vi "Load Scan.vi"(8 "error in (no error)":errorcluster, 9 "File IO.lvclass":refnum<class "File IO.lvclass">, 10 "Reader.lvclass":refnum<class "Reader.lvclass">, 11 "Scanner.lvclass":refnum<class "Scanner.lvclass">) -> (0 "error out":errorcluster, 1 "File IO.lvclass out":refnum<class "File IO.lvclass">, 2 "Reader.lvclass out":refnum<class "Reader.lvclass">, 3 "Scanner.lvclass out":refnum<class "Scanner.lvclass">)   [LabVIEW 2012, in "File IO.lvclass"]
uses:
  File IO.lvclass
  Scanners/Scanner/Scanner.lvclass
  Readers/Reader/Reader.lvclass
  Global/File Locations.vi
  Main/Scan Driver/Settings Panel.vi
  Scanners/Scanner/Write Range UI.vi
  <vilib>/Utility/file.llb/Read From Spreadsheet File (string).vi
  <vilib>/Utility/file.llb/Read From Spreadsheet File (I64).vi
  Readers/Reader/Setup UI.vi
  Main/Scan Driver/Scan Driver.lvclass
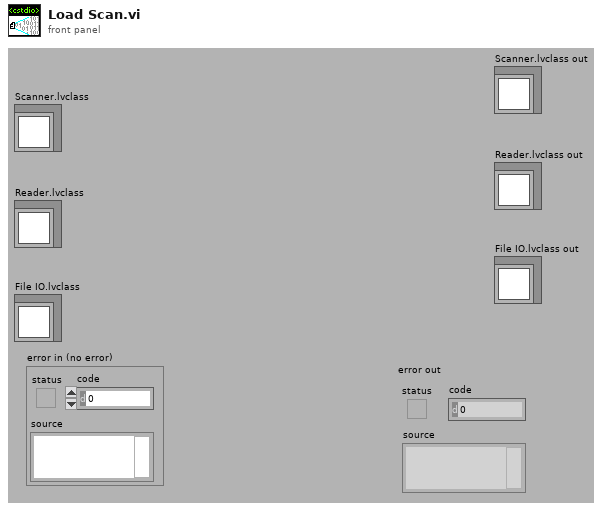
[diagram p1: front panel]
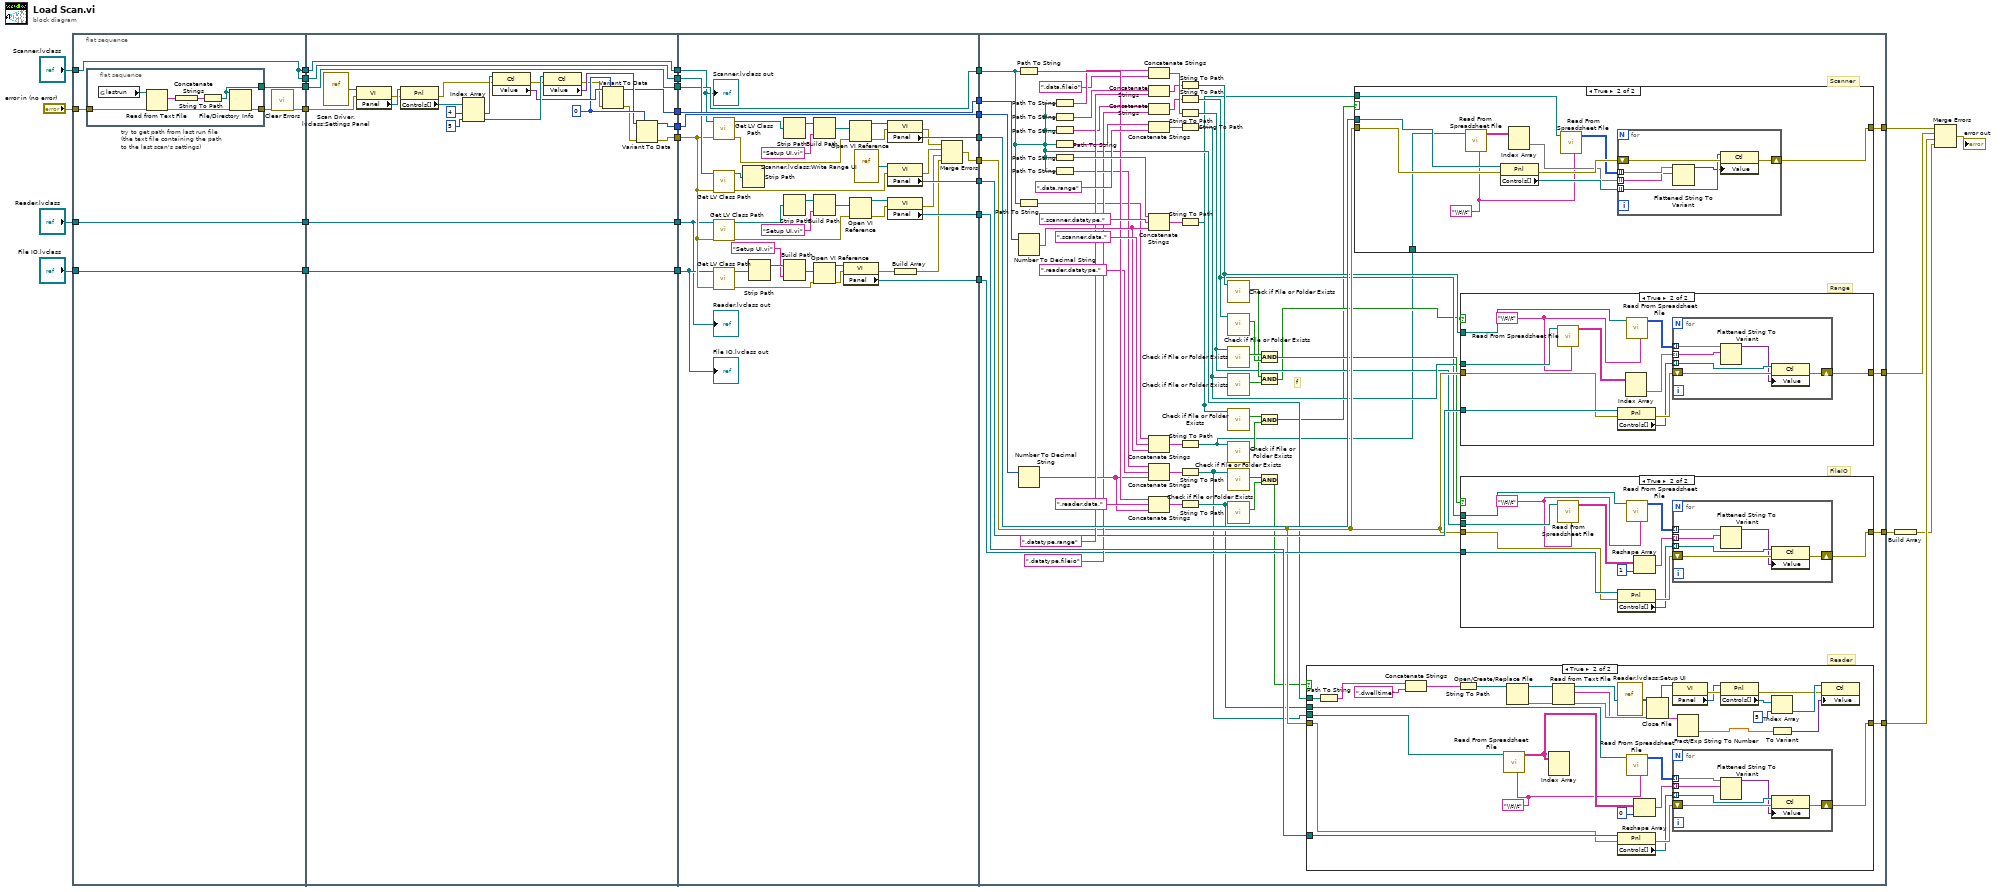
[diagram p0: block diagram]
diagram:
  n1 = flat-sequence {
    tunnel: "Scanner.lvclass" -> [w39]
    tunnel: "error in (no error)" -> [w37]
    tunnel: "Reader.lvclass" -> [w38]
    tunnel: "File IO.lvclass" -> [w33]
    tunnel: [w33] -> w32
    tunnel: [w39] -> w31
    tunnel: [w39] -> w30
    tunnel: [w38] -> w29
    tunnel: [w36] -> w28
    tunnel: [w34] -> w27
    tunnel: w32 -> [w48]
    tunnel: [w48] -> w26
    tunnel: [w70] -> w25
    tunnel: [w69] -> w24
    tunnel: [w68] -> w23
    tunnel: [w52] -> w22
    tunnel: [w51] -> w21
    tunnel: [w50] -> w20
    tunnel: w31 -> [w68]
    tunnel: w30 -> [w69]
    tunnel: w29 -> [w70]
    tunnel: [w49] -> w19
    tunnel: w28 -> [w49]
    tunnel: w27 -> [w47]
    tunnel: w26 -> [w74]
    tunnel: w25 -> [w71]
    tunnel: w24 -> [w103]
    tunnel: w23 -> [w75]
    tunnel: w22 -> [w90]
    tunnel: w21 -> [w112]
    tunnel: [w112] -> w18
    tunnel: w20 -> [w111]
    tunnel: [w111] -> w17
    tunnel: [w105] -> w16
    tunnel: [w102] -> w15
    tunnel: [w96] -> w14
    tunnel: [w89] -> w13
    tunnel: [w77] -> w12
    tunnel: w19 -> [w76]
    tunnel: [w76] -> w11
    tunnel: w18 -> [w165]
    tunnel: w17 -> [w164]
    tunnel: w16 -> [w162]
    tunnel: w15 -> [w156]
    tunnel: w14 -> [w149]
    tunnel: w13 -> [w142]
    tunnel: w12 -> [w134]
    tunnel: w11 -> [w120]
    tunnel: [w141] -> w6
    tunnel: [w140] -> w5
    tunnel: [w139] -> w4
    tunnel: [w138] -> w2
    frame #0 {
      n2 = flat-sequence "try to get path from last run file\n(the text file containing the path\nto the last scan's settings)" {
        tunnel: [w44] -> w35
        tunnel: w37 -> [w41]
        tunnel: [w40] -> w36
        frame #0 {
          n3 = global read "File Locations.vi" "lastrun"() -> (w46:path)
          n4 = Read from Text File(file (use dialog)=w46, error in=w41) -> (text=w43:string, error out=w45:errorcluster)  [unwired: 4 out]
          n5 = Concatenate Strings(w43) -> (w42:string)
          n6 = String To Path(string=w42) -> (path=w40:path)
          n7 = File/Directory Info(path=w40, error in=w45) -> (error out=w44:errorcluster)  [unwired: 6 out]
        }
      }
      n8 = call <vilib>:"Clear Errors.vi"("error in (no error)"=w35) -> ("error out"=w34:errorcluster)  [unwired: 6 in]
    }
    frame #1 {
      w59 = 0
      n9 = vi-ref "Scan Driver.lvclass:Settings Panel.vi"() -> (w67:refnum<vi>)
      n10 = property class="VI"(reference=w67, error in=w47) -> (error out=w57:errorcluster, "Panel"=w66:refnum<vi>)  [unwired: 1 out]
      n11 = property class="Pnl"(reference=w66, error in=w57) -> (error out=w56:errorcluster, "Controls[]"=w65:refnum<vi>[])  [unwired: 1 out]
      n12 = Index Array(array=w65, index #1=4, index #2=5) -> (element #1=w64:refnum<vi>, element #2=w61:refnum<vi>)
      n13 = property class="Ctl"(reference=w64, error in=w56) -> (error out=w55:errorcluster, "Value"=w60:variant)  [unwired: 1 out]
      n14 = property class="Ctl"(reference=w61, error in=w55) -> (error out=w54:errorcluster, "Value"=w58:variant)  [unwired: 1 out]
      n15 = Variant To Data(error in=w54, type=w59, Variant=w60) -> (data=w51:i32, error out=w53:errorcluster)
      n16 = Variant To Data(error in=w53, type=w59, Variant=w58) -> (data=w50:i32, error out=w52:errorcluster)
    }
    frame #2 {
      n17 = call <vilib>:"Get LV Class Path.vi"("error in (no error)"=w90, "object"=w75) -> ("error out"=w86:errorcluster, "class path"=w110:path)  [unwired: 8 out]
      n18 = call <vilib>:"Get LV Class Path.vi"("error in (no error)"=w90, "object"=w103) -> ("error out"=w73:errorcluster, "class path"=w104:path)  [unwired: 8 out]
      n19 = call <vilib>:"Get LV Class Path.vi"("error in (no error)"=w90, "object"=w71) -> ("error out"=w84:errorcluster, "class path"=w101:path)  [unwired: 8 out]
      n20 = call <vilib>:"Get LV Class Path.vi"("error in (no error)"=w90, "object"=w74) -> ("error out"=w78:errorcluster, "class path"=w95:path)  [unwired: 8 out]
      n21 = Strip Path(path=w104) -> ()  [unwired: 2 out]
      n22 = Strip Path(path=w95) -> (stripped path=w94:path)  [unwired: 1 out]
      n23 = Strip Path(path=w110) -> (stripped path=w109:path)  [unwired: 1 out]
      n24 = Strip Path(path=w101) -> (stripped path=w100:path)  [unwired: 1 out]
      n25 = Build Path(base path=w94, name or relative path="Setup UI.vi") -> (appended path=w92:path)
      n26 = Build Path(base path=w109, name or relative path="Setup UI.vi") -> (appended path=w107:path)
      n27 = Build Path(base path=w100, name or relative path="Setup UI.vi") -> (appended path=w98:path)
      n28 = Open VI Reference(vi path=w92, error in (no error)=w78) -> (vi reference=w91:refnum<vi>, error out=w79:errorcluster)  [unwired: 4 out]
      n29 = property class="VI"(reference=w91, error in=w79) -> (error out=w80:errorcluster, "Panel"=w89:refnum<vi>)  [unwired: 1 out]
      n30 = Open VI Reference(vi path=w107, error in (no error)=w86) -> (vi reference=w106:refnum<vi>, error out=w87:errorcluster)  [unwired: 4 out]
      n31 = Open VI Reference(vi path=w98, error in (no error)=w84) -> (vi reference=w97:refnum<vi>, error out=w83:errorcluster)  [unwired: 4 out]
      n32 = vi-ref "Scanner.lvclass:Write Range UI.vi"() -> (w72:refnum<vi>)
      n33 = property class="VI"(reference=w106, error in=w87) -> (error out=w88:errorcluster, "Panel"=w105:refnum<vi>)  [unwired: 1 out]
      n34 = property class="VI"(reference=w72, error in=w73) -> (error out=w85:errorcluster, "Panel"=w102:refnum<vi>)  [unwired: 1 out]
      n35 = property class="VI"(reference=w97, error in=w83) -> (error out=w82:errorcluster, "Panel"=w96:refnum<vi>)  [unwired: 1 out]
      n36 = Build Array(w80) -> (w81:errorcluster[])
      n37 = Merge Errors(w88, w85, w82, w81) -> (w77:errorcluster)
      "Scanner.lvclass out" <- w75
      "Reader.lvclass out" <- w71
      "File IO.lvclass out" <- w74
    }
    frame #3 {
      # "f"
      # "FileIO"
      # "Reader"
      # "Range"
      # "Scanner"
      n38 = Path To String(path=w120) -> (string=w155:string)
      n39 = Path To String(path=w120) -> (string=w137:string)
      n40 = Number To Decimal String(number=w165) -> (decimal integer string=w163:string)  [unwired: 1 in]
      n41 = Number To Decimal String(number=w164) -> (decimal integer string=w148:string)  [unwired: 1 in]
      n42 = Path To String(path=w120) -> (string=w147:string)
      n43 = Path To String(path=w120) -> (string=w158:string)
      n44 = Path To String(path=w120) -> (string=w144:string)
      n45 = Path To String(path=w120) -> (string=w161:string)
      n46 = Path To String(path=w120) -> (string=w168:string)
      n47 = Path To String(path=w120) -> (string=w152:string)
      n48 = Concatenate Strings(w147, ".data.fileio") -> (w145:string)
      n49 = Concatenate Strings(w158, ".datatype.range") -> (w135:string)
      n50 = Concatenate Strings(w144, ".datatype.fileio") -> (w136:string)
      n51 = Concatenate Strings(w161, ".data.range") -> (w159:string)
      n52 = Concatenate Strings(w168, ".scanner.datatype.", w163) -> (w166:string)
      n53 = Concatenate Strings(w137, ".scanner.data.", w163) -> (w169:string)
      n54 = Concatenate Strings(w152, ".reader.datatype.", w148) -> (w150:string)
      n55 = Concatenate Strings(w155, ".reader.data.", w148) -> (w153:string)
      n56 = String To Path(string=w135) -> (path=w124:path)
      n57 = String To Path(string=w136) -> (path=w122:path)
      n58 = String To Path(string=w145) -> (path=w121:path)
      n59 = String To Path(string=w159) -> (path=w123:path)
      n60 = String To Path(string=w166) -> (path=w116:path)
      n61 = String To Path(string=w169) -> (path=w115:path)
      n62 = String To Path(string=w150) -> (path=w113:path)
      n63 = String To Path(string=w153) -> (path=w114:path)
      n64 = call <vilib>:"Check if File or Folder Exists.vi"("path"=w124) -> ("file or folder exists?"=w130:bool)  [unwired: 8 in, 2 out]
      n65 = call <vilib>:"Check if File or Folder Exists.vi"("path"=w122) -> ("file or folder exists?"=w132:bool)  [unwired: 8 in, 2 out]
      n66 = call <vilib>:"Check if File or Folder Exists.vi"("path"=w121) -> ("file or folder exists?"=w133:bool)  [unwired: 8 in, 2 out]
      n67 = call <vilib>:"Check if File or Folder Exists.vi"("path"=w123) -> ("file or folder exists?"=w129:bool)  [unwired: 8 in, 2 out]
      n68 = call <vilib>:"Check if File or Folder Exists.vi"("path"=w116) -> ("file or folder exists?"=w128:bool)  [unwired: 8 in, 2 out]
      n69 = call <vilib>:"Check if File or Folder Exists.vi"("path"=w115) -> ("file or folder exists?"=w127:bool)  [unwired: 8 in, 2 out]
      n70 = call <vilib>:"Check if File or Folder Exists.vi"("path"=w113) -> ("file or folder exists?"=w126:bool)  [unwired: 8 in, 2 out]
      n71 = call <vilib>:"Check if File or Folder Exists.vi"("path"=w114) -> ("file or folder exists?"=w125:bool)  [unwired: 8 in, 2 out]
      n72 = And(x=w133, y=w132) -> (x .and. y?=w131:bool)
      n73 = And(x=w130, y=w129) -> (x .and. y?=w118:bool)
      n74 = And(x=w128, y=w127) -> (x .and. y?=w117:bool)
      n75 = And(x=w126, y=w125) -> (x .and. y?=w119:bool)
      n76 = case shown="True" w119 {
        tunnel: w149 -> [_ w238]
        tunnel: [w207 w237] -> w139
        tunnel: w134 -> [w207 w236]
        tunnel: w114 -> [_ w235]
        tunnel: w113 -> [_ w234]
        tunnel: w120 -> [_ w233]
        frame False {
        }
        frame True {
          w208 = "\\t\\t"
          n77 = Path To String(path=w233) -> (string=w228:string)
          n78 = Concatenate Strings(w228, ".dwelltime") -> (w226:string)
          n79 = String To Path(string=w226) -> (path=w225:path)
          n80 = call-poly <vilib>:"Read From Spreadsheet File.vi"("delimiter (\\t)"=w208, "file path (dialog if empty)"=w234) -> ("all rows"=w211:string[][])  [unwired: 5 in, 4 out]
          n81 = Open/Create/Replace File(file path (use dialog)=w225) -> (refnum out=w230:refnum<file>, error out=w232:errorcluster)  [unwired: 5 in, 1 out]
          n82 = Index Array(array=w211) -> ()  [unwired: 2 in, 1 out]
          n83 = Read from Text File(file (use dialog)=w230, error in=w232) -> (refnum out=w231:refnum<file>, text=w224:string, error out=w229:errorcluster)  [unwired: 2 in, 1 out]
          n84 = vi-ref "Reader.lvclass:Setup UI.vi"() -> (w223:refnum<vi>)
          n85 = property class="Pnl"(reference=w238, error in=w236) -> (error out=w214:errorcluster, "Controls[]"=w213:refnum<vi>[])  [unwired: 1 out]
          n86 = call-poly <vilib>:"Read From Spreadsheet File.vi"("delimiter (\\t)"=w208, "file path (dialog if empty)"=w235) -> ("all rows"=w212:i64[][])  [unwired: 5 in, 4 out]
          n87 = Reshape Array(w211, 0) -> (w209:string[])
          n88 = Close File(refnum=w231, error in=w229) -> ()  [unwired: 2 out]
          n89 = property class="VI"(reference=w223) -> (error out=w222:errorcluster, "Panel"=w221:refnum<vi>)  [unwired: 1 in, 1 out]
          n90 = for {
            shift-right: [w243] -> w237
            shift-left: w214 -> [w244]
            tunnel: w213 -> [w242] mode=indexing
            tunnel: w212 -> [w240] mode=indexing
            tunnel: w209 -> [w239] mode=indexing
            n91 = Flattened String To Variant(6:w239, 7:w240) -> (3:w241:variant)  [unwired: 1 in, 1 out]
            n92 = property class="Ctl"(reference=w242, error in=w244, "Value"=w241) -> (error out=w243:errorcluster)  [unwired: 1 out]
          }
          n93 = Fract/Exp String To Number(string=w224) -> (number=w216:dbl)  [unwired: 3 in, 1 out]
          n94 = property class="Pnl"(reference=w221, error in=w222) -> (error out=w218:errorcluster, "Controls[]"=w220:refnum<vi>[])  [unwired: 1 out]
          n95 = Index Array(array=w220, index=5) -> (element=w219:refnum<vi>)
          n96 = To Variant(anything=w216) -> (Variant=w215:variant)
          n97 = property class="Ctl"(reference=w219, error in=w218, "Value"=w215) -> ()  [unwired: 2 out]
        }
      }
      n98 = case shown="True" w117 {
        tunnel: w162 -> [_ w182]
        tunnel: [w171 w181] -> w141
        tunnel: w134 -> [w171 w180]
        tunnel: w116 -> [_ w173]
        tunnel: w115 -> [_ w172]
        frame False {
        }
        frame True {
          w174 = "\\t\\t"
          n99 = call-poly <vilib>:"Read From Spreadsheet File.vi"("delimiter (\\t)"=w174, "file path (dialog if empty)"=w172) -> ("all rows"=w176:string[][])  [unwired: 5 in, 4 out]
          n100 = property class="Pnl"(reference=w182, error in=w180) -> (error out=w179:errorcluster, "Controls[]"=w178:refnum<vi>[])  [unwired: 1 out]
          n101 = Index Array(array=w176) -> (element=w175:string[])  [unwired: 2 in]
          n102 = call-poly <vilib>:"Read From Spreadsheet File.vi"("delimiter (\\t)"=w174, "file path (dialog if empty)"=w173) -> ("all rows"=w177:i64[][])  [unwired: 5 in, 4 out]
          n103 = for {
            shift-right: [w187] -> w181
            shift-left: w179 -> [w188]
            tunnel: w178 -> [w186] mode=indexing
            tunnel: w177 -> [w184] mode=indexing
            tunnel: w175 -> [w183] mode=indexing
            n104 = Flattened String To Variant(6:w183, 7:w184) -> (3:w185:variant)  [unwired: 1 in, 1 out]
            n105 = property class="Ctl"(reference=w186, error in=w188, "Value"=w185) -> (error out=w187:errorcluster)  [unwired: 1 out]
          }
        }
      }
      n106 = case shown="True" w118 {
        tunnel: w156 -> [_ w200]
        tunnel: [w189 w199] -> w140
        tunnel: w134 -> [w189 w193]
        tunnel: w124 -> [_ w192]
        tunnel: w123 -> [_ w191]
        frame False {
        }
        frame True {
          w190 = "\\t\\t"
          n107 = call-poly <vilib>:"Read From Spreadsheet File.vi"("delimiter (\\t)"=w190, "file path (dialog if empty)"=w191) -> ("all rows"=w196:string[][])  [unwired: 5 in, 4 out]
          n108 = property class="Pnl"(reference=w200, error in=w193) -> (error out=w198:errorcluster, "Controls[]"=w197:refnum<vi>[])  [unwired: 1 out]
          n109 = Index Array(array=w196) -> (element=w195:string[])  [unwired: 2 in]
          n110 = call-poly <vilib>:"Read From Spreadsheet File.vi"("delimiter (\\t)"=w190, "file path (dialog if empty)"=w192) -> ("all rows"=w194:i64[][])  [unwired: 5 in, 4 out]
          n111 = for {
            shift-right: [w205] -> w199
            shift-left: w198 -> [w206]
            tunnel: w197 -> [w204] mode=indexing
            tunnel: w195 -> [w202] mode=indexing
            tunnel: w194 -> [w201] mode=indexing
            n112 = Flattened String To Variant(6:w202, 7:w201) -> (3:w203:variant)  [unwired: 1 in, 1 out]
            n113 = property class="Ctl"(reference=w204, error in=w206, "Value"=w203) -> (error out=w205:errorcluster)  [unwired: 1 out]
          }
        }
      }
      n114 = case shown="True" w131 {
        tunnel: w142 -> [_ w257]
        tunnel: [w245 w256] -> w138
        tunnel: w134 -> [w245 w255]
        tunnel: w122 -> [_ w254]
        tunnel: w121 -> [_ w253]
        frame False {
        }
        frame True {
          w249 = "\\t\\t"
          n115 = call-poly <vilib>:"Read From Spreadsheet File.vi"("delimiter (\\t)"=w249, "file path (dialog if empty)"=w253) -> ("all rows"=w248:string[][])  [unwired: 5 in, 4 out]
          n116 = property class="Pnl"(reference=w257, error in=w255) -> (error out=w252:errorcluster, "Controls[]"=w251:refnum<vi>[])  [unwired: 1 out]
          n117 = call-poly <vilib>:"Read From Spreadsheet File.vi"("delimiter (\\t)"=w249, "file path (dialog if empty)"=w254) -> ("all rows"=w250:i64[][])  [unwired: 5 in, 4 out]
          n118 = Reshape Array(w248, 1) -> (w246:string[])
          n119 = for {
            shift-right: [w262] -> w256
            shift-left: w252 -> [w263]
            tunnel: w251 -> [w261] mode=indexing
            tunnel: w250 -> [w259] mode=indexing
            tunnel: w246 -> [w258] mode=indexing
            n120 = Flattened String To Variant(6:w258, 7:w259) -> (3:w260:variant)  [unwired: 1 in, 1 out]
            n121 = property class="Ctl"(reference=w261, error in=w263, "Value"=w260) -> (error out=w262:errorcluster)  [unwired: 1 out]
          }
        }
      }
    }
  }
  n122 = Build Array(w2) -> (w3:errorcluster[])
  n123 = Merge Errors(w6, w5, w4, w3) -> (→"error out":errorcluster)
